vi "Mark Active.vi"(9 "Round":i32, 10 "Idx":i32, 11 "Board":refnum<data-value>) -> ()   [LabVIEW 2015, in "Formation.lvclass"]
uses:
  Formation.lvclass
  Board Cluster.ctl
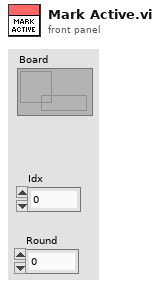
[diagram p1: front panel]
types:
  T1 = typedef "Formation.lvclass/Board Cluster.ctl" = cluster{"Board S":i32, "Pos[Idx]":cluster{"X":i32, "Y":i32}[], "Round[Idx]":i32[]}
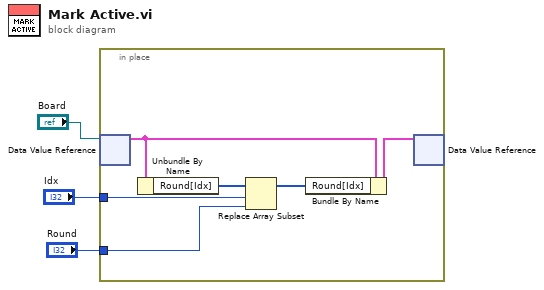
[diagram p0: block diagram]
diagram:
  n1 = in-place {
    in-place-border: "Idx" -> [w8]
    in-place-border: "Round" -> [w7]
    n2 = in-place-dvr #1("Board") -> (w6:T1)  [unwired: 1 out]
    n3 = Unbundle By Name(w6) -> ("Round[Idx]"=w9:i32[])
    n4 = Replace Array Subset(array=w9, new element=w7, index=w8) -> (w5:i32[])
    n5 = Bundle By Name(cluster=w6, "Round[Idx]"=w5) -> (w4:T1)
    n6 = in-place-dvr #1(w4) -> ()  [unwired: 2 out]
  }
